vi "Template.vi"() -> ()   [LabVIEW 2010]
uses:
  lib/Ports.lvclass
panel:
  in  "DigNum Refnum":refnum<vi>
  out "Состояни процессов":string[][](table)
  in  "OUT Ports Array":cluster{"String":string, "Array 2":bool[]}[](array[cluster])
  in  "INP Ports Array":cluster{"String":string, "Array 2":bool[]}[](array[cluster])
  in  "Значения выходных глобальных переменных":string[][](table)
  in  "Значения входных глобальных переменных":string[][](table)
  out "Выходжные сообщения":string[][](table)
  in  "Open code Editor":bool
  # "Алгоритм управления"
  # "Значения входных портов"
  # "Значения выходных портов"
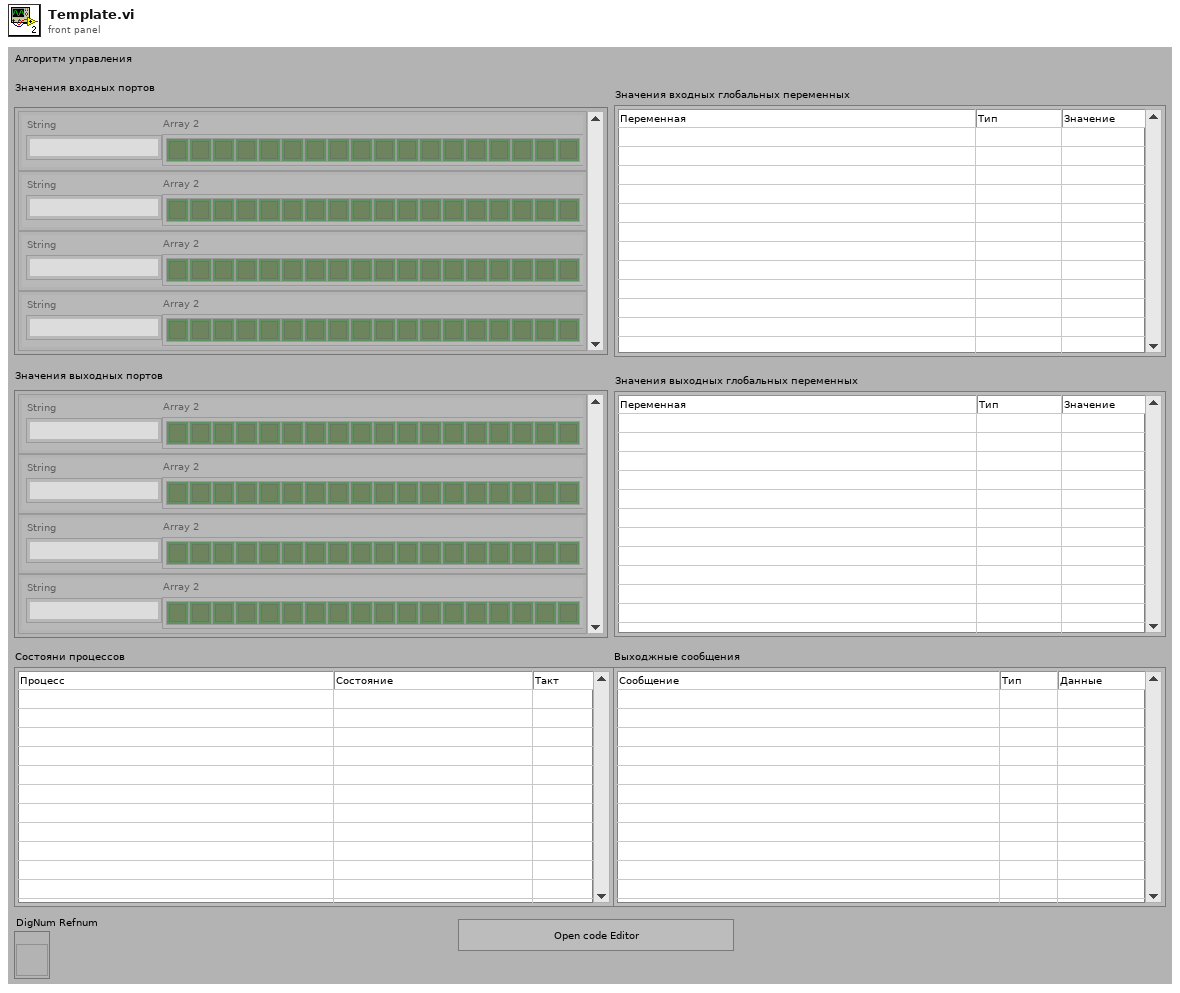
[diagram p1: front panel]
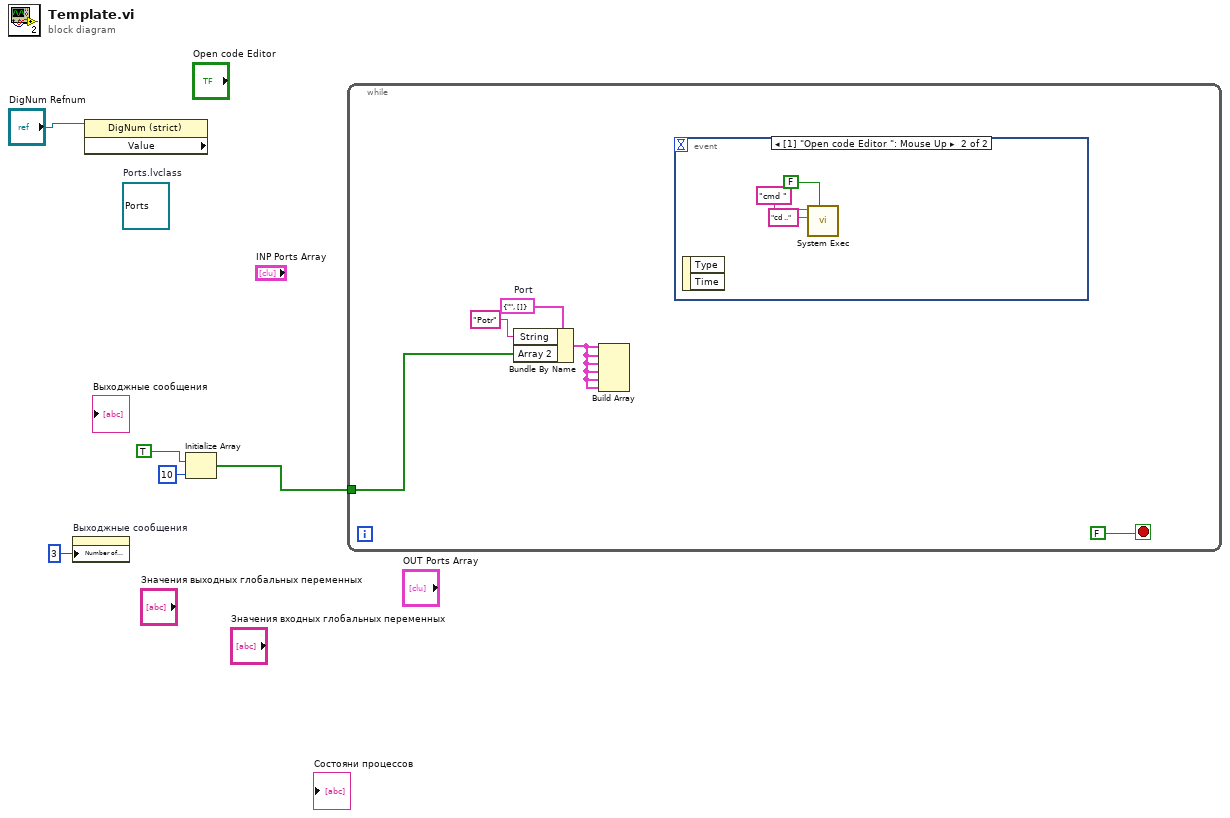
[diagram p0: block diagram]
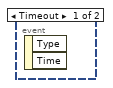
[diagram p2: hidden frame]
diagram:
  (unwired) refnum<class "Ports.lvclass"> refnum  # Ports.lvclass
  n1 = property on="Выходжные сообщения" class="Tbl (strict)"("Number of Columns"=u32 3 ("Number of Rows")) -> ()  [unwired: 2 in, 2 out]
  n2 = property class="DigNum (strict)" props=["Value"](reference="DigNum Refnum") -> ()  [unwired: 1 in, 3 out]
  n3 = Initialize Array(TRUE ("Boolean"), 10 ("dimension size")) -> (w3:bool[])
  n4 = while {
    tunnel: w3 -> [w7]
    stop <- FALSE ("stop") stop-if-true
    w8 = cluster{"String":string, "Array 2":bool[]} {"String"="", "Array 2"=[]}  # Port
    n5 = Bundle By Name(cluster=w8, "String"="Potr", "Array 2"=w7) -> (w6:cluster{"String":string, "Array 2":bool[]})
    n6 = Build Array(w6, w6, w6, w6, w6, w6) -> ()  [unwired: 1 out]
    n7 = event shown="[1] \"Open code Editor \": Mouse Up" {
      selector: _ -> [_ _]
      dyn-events: _ -> [_ _]
      timeout: _ -> [_ _]
      event Timeout {
        n8 = event-data() -> ()  [unwired: 1 in, 2 out]
      }
      event "Open code Editor": Mouse Up {
        n9 = event-data() -> ()  [unwired: 1 in, 2 out]
        n10 = call <vilib>:"System Exec.vi"("wait until completion? (T)"=FALSE, "standard input"="cd ..", "command line"="cmd ") -> ()  [unwired: 5 in, 4 out]
      }
    }
  }
